vi "Out_S9F13.vi"(8 "error in (no error)":errorcluster, 9 "EDID":string, 10 "MEXP":string, 11 "S9 Message Class in":refnum<class "S9 Message Class.lvclass">) -> (0 "error out":errorcluster, 3 "S9 Message Class out":refnum<class "S9 Message Class.lvclass">)   [LabVIEW 2020, in "SECS Communication.lvlib" / "S9 Message Class.lvclass"]
uses:
  S9 Message Class.lvclass
  D:/Dropbox/SECS/SECS_GEM v1.1.0/Com/SECS Communication/SECS-II Class/SECS-II Class.lvclass
  SECS-II Class/Data Message_List.vi
  SECS-II Class/Data Message_ASCII.vi
  SECS-II Class/SECS-II Class.lvclass
  D:/Dropbox/SECS/SECS_GEM v1.1.0/Com/SECS Communication/S9 Message Class/S9 Message Class.lvclass
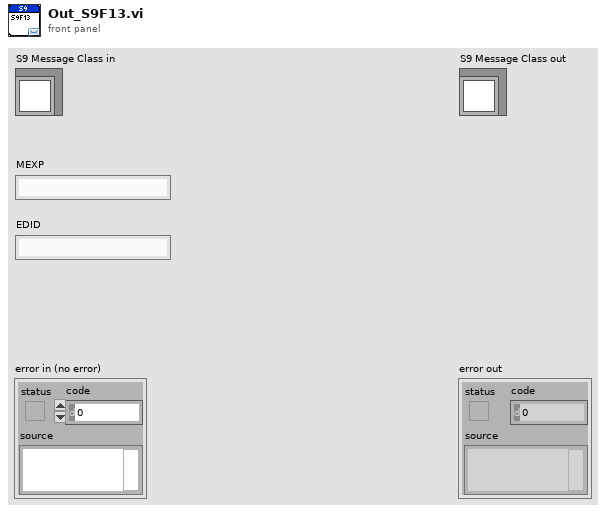
[diagram p1: front panel]
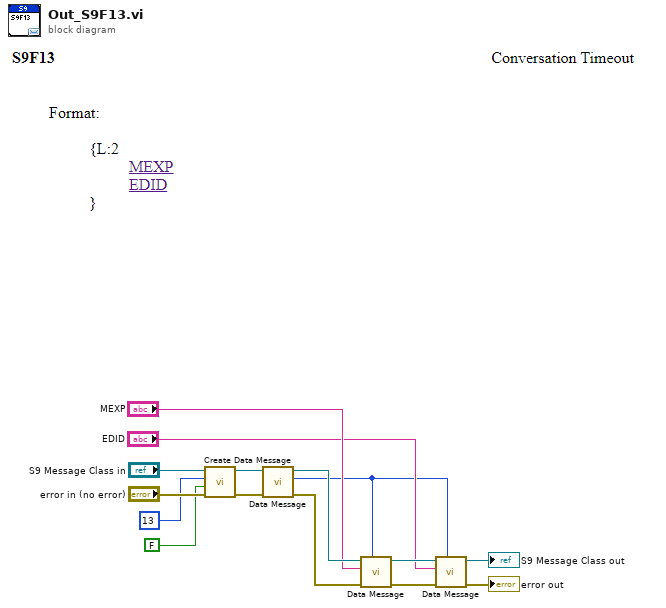
[diagram p0: block diagram]
diagram:
  n1 = call "Create Data Message.vi"("error in (no error)"="error in (no error)", "W-Bit"=FALSE, "Function"=u8 13, "SECS-II Class in"="S9 Message Class in") -> ("error out"=w11:errorcluster, "SECS-II Class out"=w10:refnum<class "S9 Message Class.lvclass">)  [unwired: 6 in]
  n2 = call-poly "Data Message.vi"("error in"=w11, "SECS-II Class in"=w10) -> ("error out"=w9:errorcluster, "Index"=w1:i32, "SECS-II Class out"=w8:refnum<class "S9 Message Class.lvclass">)  [unwired: 7 in]
  n3 = call-poly "Data Message.vi"("Parent Index"=w1, "error in"=w9, "Data"="MEXP", "SECS-II Class in"=w8) -> ("error out"=w6:errorcluster, "SECS-II Class out"=w7:refnum<class "S9 Message Class.lvclass">)  [unwired: 6 in]
  n4 = call-poly "Data Message.vi"("Parent Index"=w1, "error in"=w6, "Data"="EDID", "SECS-II Class in"=w7) -> ("error out"=→"error out":errorcluster, "SECS-II Class out"=→"S9 Message Class out":refnum<class "S9 Message Class.lvclass">)  [unwired: 6 in]
